vi "WriteRead.vi"(6 "Timeout (ms)":i32=1000, 8 "error in (no error)":errorcluster, 9 "warn?":bool=TRUE, 10 "String in":string, 11 "VISA Refnum in":refnum<visa-resource-name>) -> (0 "error out":errorcluster, 1 "warned":bool, 2 "String out":string, 3 "VISA Refnum out":refnum<visa-resource-name>)   [LabVIEW 2023]
uses:
  ShapekoGlobal.vi
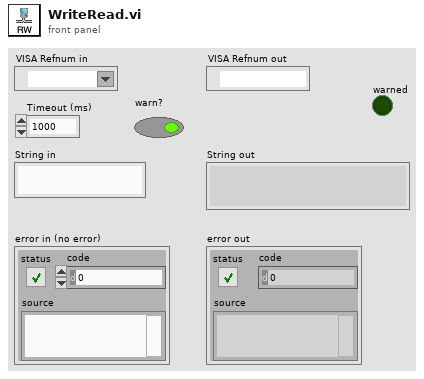
[diagram p1: front panel]
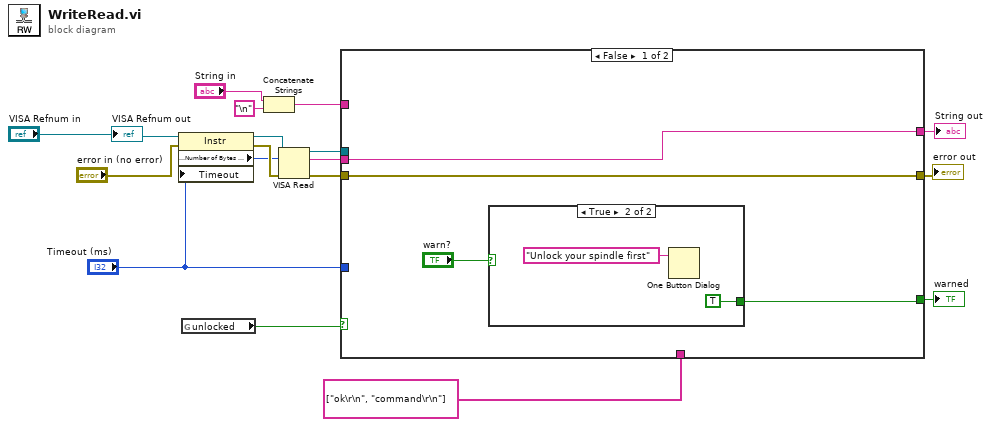
[diagram p0: block diagram]
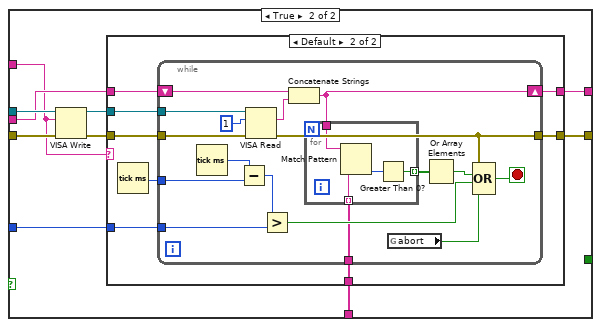
[diagram p3: hidden frame]
diagram:
  n1 = property class="Instr"(reference="VISA Refnum in", error in="error in (no error)", "Timeout"="Timeout (ms)") -> (reference out=w11:refnum<visa-resource-name>, error out=w13:errorcluster, "Serial Settings:Number of Bytes at Serial Port"=w12:u32)
  n2 = global read "ShapekoGlobal.vi" "unlocked"() -> (w4:bool)
  n3 = Concatenate Strings("String in", "\n" ("string")) -> (w6:string)
  n4 = VISA Read(VISA resource name=w11, byte count=w12, error in (no error)=w13) -> (VISA resource name out=w10:refnum<visa-resource-name>, read buffer=w7:string, error out=w8:errorcluster)  [unwired: 1 out]
  n5 = case shown="False" w4 {
    tunnel: [w21 w33] -> w17
    tunnel: [w20 w30] -> w16
    tunnel: w10 -> [_ w29]
    tunnel: w8 -> [w20 w28]
    tunnel: w7 -> [w21 w27]
    tunnel: "Timeout (ms)" -> [_ w26]
    tunnel: w6 -> [_ w25]
    tunnel: string[] ["ok\r\n", "command\r\n"] -> [_ w24]
    tunnel: [w18 _] -> w1
    frame False {
      n6 = case shown="True" "warn?" {
        tunnel: [_ TRUE] -> w18
        frame False {
        }
        frame True {
          n7 = One Button Dialog(message="Unlock your spindle first") -> ()  [unwired: 1 in, 1 out]
        }
      }
    }
    frame True {
      n8 = VISA Write(VISA resource name=w29, write buffer=w25, error in (no error)=w28) -> (VISA resource name out=w31:refnum<visa-resource-name>, error out=w32:errorcluster)  [unwired: 1 out]
      n9 = case shown="Default" w25 {
        tunnel: [w35 w43] -> w33
        tunnel: w32 -> [w34 w42]
        tunnel: w31 -> [_ w41]
        tunnel: [w34 w40] -> w30
        tunnel: w27 -> [w35 w39]
        tunnel: w26 -> [_ w38]
        tunnel: w24 -> [_ w36]
        frame "" {
        }
        frame Default {
          n10 = Tick Count (ms)() -> (millisecond timer value=w37:u32)
          n11 = while {
            tunnel: w41 -> [w60]
            tunnel: w42 -> [w59]
            shift-right: [w56] -> w43
            shift-left: w39 -> [w58]
            tunnel: [w48] -> w40
            tunnel: w37 -> [w53]
            tunnel: w38 -> [w51]
            tunnel: w36 -> [w46]
            stop <- w49 stop-if-true
            n12 = Tick Count (ms)() -> (millisecond timer value=w54:u32)
            n13 = Subtract(x=w54, y=w53) -> (x-y=w52:u32)
            n14 = VISA Read(VISA resource name=w60, byte count=u32 1, error in (no error)=w59) -> (read buffer=w57:string, error out=w48:errorcluster)  [unwired: 2 out]
            n15 = Greater?(x=w52, y=w51) -> (0:w50:bool)
            n16 = Concatenate Strings(w58, w57) -> (w56:string)
            n17 = for {
              tunnel: w56 -> [w64]
              tunnel: [w62] -> w47 mode=indexing
              tunnel: w46 -> [w61] mode=indexing
              n18 = Match Pattern(string=w64, regular expression=w61) -> (offset past match=w63:i32)  [unwired: 1 in, 3 out]
              n19 = Greater Than 0?(x=w63) -> (x > 0?=w62:bool)
            }
            n20 = global read "ShapekoGlobal.vi" "abort"() -> (w44:bool)
            n21 = Or Array Elements(Boolean array=w47) -> (logical OR=w45:bool)
            n22 = Compound Arithmetic op=OR(w48, w45, w50, w44) -> (w49:bool)
          }
        }
      }
    }
  }
  "String out" <- w17
  "error out" <- w16
  "warned" <- w1
  "VISA Refnum out" <- "VISA Refnum in"
